vi "LV Graphs to Igor Example.vi"() -> ()   [LabVIEW 2019, in "LV-Data.ITX.lvclass"]
uses:
  LV-Data.ITX.lvclass
  <userlib>/LevyLab/Graph Utilities/graph_utilities.lvclass/graph_utilities.ctl
  <userlib>/LevyLab/XY Utilities/subVIs/Multiply float (multiple).vi
  <userlib>/LevyLab/Graph Utilities/XY Graph/Set XY Graph Value (array).vi
  <userlib>/LevyLab/Graph Utilities/XY Graph/Get XY Graph Value.vi
  <userlib>/LevyLab/XY Utilities/XY to 2D.vi
  <userlib>/LevyLab/Graph Utilities/Intensity Graph/Set Intensity Graph Value.vi
  <userlib>/LevyLab/Graph Utilities/Intensity Graph/Set Intensity Graph X Scale Array.vi
  <userlib>/LevyLab/Graph Utilities/XY Graph/Get XY Graph X Label.vi
  <userlib>/LevyLab/Graph Utilities/Intensity Graph/Set Intensity Graph X Label.vi
  <userlib>/LevyLab/Graph Utilities/XY Graph/Get XY Graph Y Label.vi
  <userlib>/LevyLab/Graph Utilities/Intensity Graph/Set Intensity Graph Z Label.vi
  <userlib>/LevyLab/Graph Utilities/Intensity Graph/Set Intensity Graph Y Scale Array.vi
  <userlib>/LevyLab/Graph Utilities/Intensity Graph/Set Intensity Graph Y Label.vi
  <userlib>/LevyLab/Graph Utilities/graph_utilities.lvclass
  <userlib>/LevyLab/XY Utilities/xy_utilities.lvlib
panel:
  out "Intensity Graph":dbl[][](graph)
  out "XY Graph":cluster{dbl[], dbl[]}[](graph)
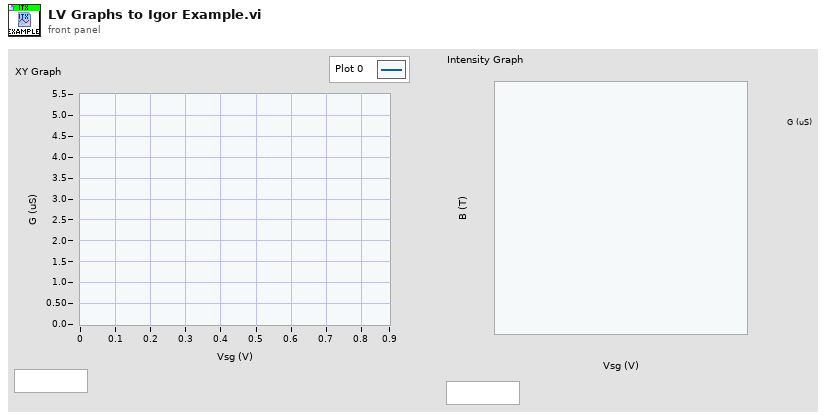
[diagram p1: front panel]
types:
  T1 = enum16{"thermal waveguide", "superlattice waveguide", "decay in atmosphere"}
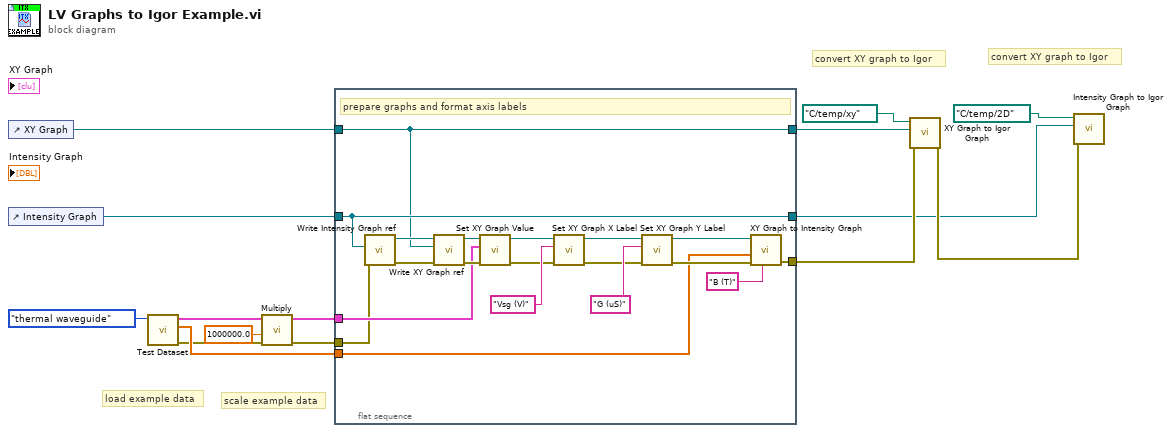
[diagram p0: block diagram]
diagram:
  # "convert XY graph to Igor"
  # "convert XY graph to Igor"
  # "scale example data"
  # "load example data"
  n1 = control-ref of="XY Graph"() -> (w10:refnum<vi>)
  n2 = control-ref of="Intensity Graph"() -> (w4:refnum<vi>)
  n3 = call <userlib>:"Test Dataset.vi"("Enum"=T1."thermal waveguide") -> ("error out"=w6:errorcluster, "Parameters out"=w11:dbl[], "XY-data out"=w13:cluster{"X-array":dbl[], "Y-array":dbl[]}[])  [unwired: 8 in]
  n4 = call-poly <userlib>:"Multiply.vi"("error in (no error)"=w6, "y (1)"=1000000.0, "XY-data"=w13) -> ("error out"=w5:errorcluster, "XY-data out"=w12:cluster{"X-array":dbl[], "Y-array":dbl[]}[])  [unwired: 7 in]
  n5 = flat-sequence {
    tunnel: w12 -> [w21]
    tunnel: w11 -> [w20]
    tunnel: w10 -> [w16]
    tunnel: [w19] -> w8
    tunnel: w5 -> [w18]
    tunnel: w4 -> [w17]
    tunnel: [w17] -> w2
    tunnel: [w16] -> w1
    frame #0 {
      # "prepare graphs and format axis labels"
      n6 = call <userlib>:"Write Intensity Graph ref.vi"("error in (no error)"=w18, "Intensity Graph"=w17) -> ("error out"=w25:errorcluster, "graph_utilities out"=w34:refnum<class "graph_utilities.lvclass">)  [unwired: 8 in]
      n7 = call <userlib>:"Write XY Graph ref.vi"("error in (no error)"=w25, "XY Graph"=w16, "graph_utilities in"=w34) -> ("error out"=w24:errorcluster, "graph_utilities out"=w33:refnum<class "graph_utilities.lvclass">)  [unwired: 7 in]
      n8 = call-poly <userlib>:"Set XY Graph Value.vi"("error in (no error)"=w24, "XY-data"=w21, "graph_utilities in"=w33) -> ("error out"=w26:errorcluster, "graph_utilities out"=w32:refnum<class "graph_utilities.lvclass">)  [unwired: 7 in]
      n9 = call <userlib>:"Set XY Graph X Label.vi"("error in (no error)"=w26, "X Label"="Vsg (V)", "graph_utilities in"=w32) -> ("error out"=w23:errorcluster, "graph_utilities out"=w31:refnum<class "graph_utilities.lvclass">)  [unwired: 7 in]
      n10 = call <userlib>:"Set XY Graph Y Label.vi"("error in (no error)"=w23, "Y Label"="G (uS)", "graph_utilities in"=w31) -> ("error out"=w22:errorcluster, "graph_utilities out"=w30:refnum<class "graph_utilities.lvclass">)  [unwired: 7 in]
      n11 = call <userlib>:"XY Graph to Intensity Graph.vi"("Y Label"="B (T)", "error in (no error)"=w22, "Y Scale"=w20, "graph_utilities in"=w30) -> ("error out"=w19:errorcluster)  [unwired: 6 in, 1 out]
    }
  }
  n12 = call "XY Graph to Igor Graph.vi"("error in (no error)"=w8, "XY Graph Reference"=w1, "Path"=path "C:/temp/xy") -> ("error out"=w7:errorcluster)  [unwired: 7 in, 1 out]
  n13 = call "Intensity Graph to Igor Graph.vi"("error in (no error)"=w7, "Intensity Graph Reference"=w2, "Path"=path "C:/temp/2D") -> ()  [unwired: 7 in, 2 out]
